vi "Read Config File.vi"(7 "LabVIEW Dir Override":path, 8 "error in (no error)":errorcluster, 10 "Config File In":string, 11 "Project Source Root":path) -> (0 "error out":errorcluster, 3 "Configuration out":T1)   [LabVIEW 2011, in "LVH-Build-Tools.lvlib"]
uses:
  LVH-Build-Tools.lvlib
  Type Defs/Configuration.ctl
  Type Defs/Install Configuration.ctl
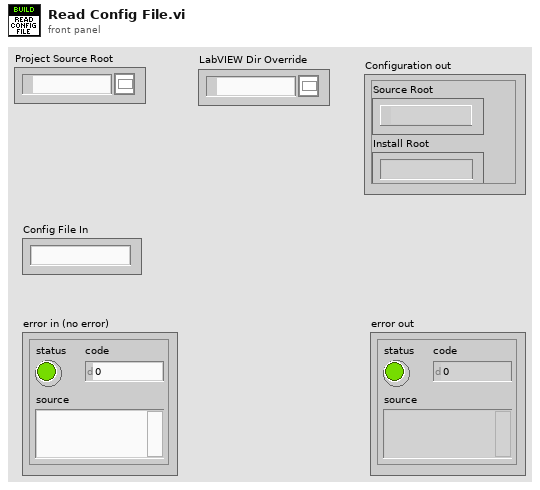
[diagram p1: front panel]
types:
  T1 = typedef "LVH-Build-Tools.lvlib/Configuration.ctl" = cluster{"Source Root":path, "Install Root":string, "Components":string[], "Ignore":string[], "Config Files":path[], "LV Directories":path[], "Install Paths":T2}
  T2 = typedef "LVH-Build-Tools.lvlib/Install Configuration.ctl" = cluster{"LabVIEW Directory":path, "Project Source Config":path}
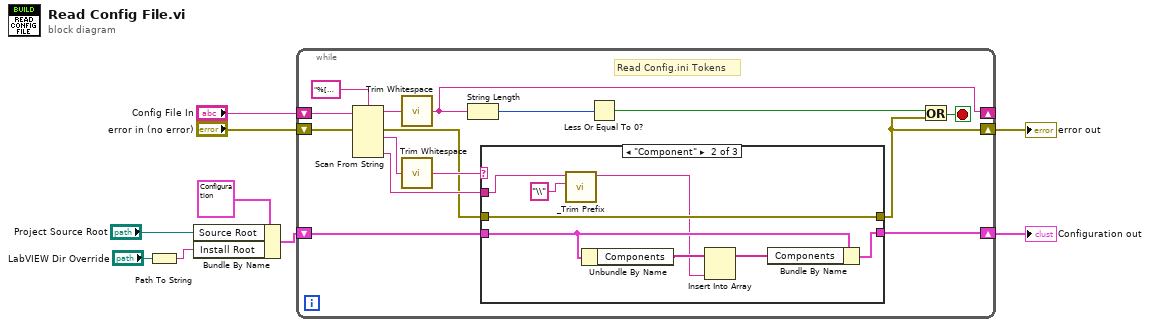
[diagram p0: block diagram]
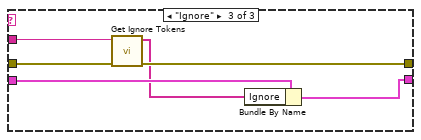
[diagram p3: hidden frame]
diagram:
  n1 = Path To String(path="LabVIEW Dir Override") -> (string=w1:string)
  n2 = Bundle By Name(cluster=T1 {"Source Root"=path "", "Install Root"="", "Components"=[], "Ignore"=[], "Config Files"=[], "LV Directories"=[], "Install Paths"={"LabVIEW Directory"=path "", "Project Source Config"=path ""}} ("Configuration in"), "Source Root"="Project Source Root", "Install Root"=w1) -> (w4:T1)
  n3 = while {
    shift-right: [w14] -> _
    shift-left: "Config File In" -> [w23]
    shift-right: [w12] -> w8
    shift-left: "error in (no error)" -> [w22]
    shift-right: [w10] -> w9
    shift-left: w4 -> [w11]
    stop <- w18 stop-if-true
    # "Read Config.ini Tokens"
    n4 = Scan From String(format string="%[^=] %[=] %[^\n]", input string=w23, error in=w22) -> (remaining string=w15:string, error out=w13:errorcluster, output 1=w17:string, output 3=w20:string)  [unwired: 5 in, 1 out]
    n5 = call <vilib>:"Trim Whitespace.vi"("string"=w15) -> ("trimmed string"=w14:string)  [unwired: 1 in]
    n6 = call <vilib>:"Trim Whitespace.vi"("string"=w17) -> ("trimmed string"=w16:string)  [unwired: 1 in]
    n7 = String Length(string=w14) -> (length=w21:i32)
    n8 = case shown="\"Component\"" w16 {
      tunnel: w20 -> [_ w29 w40]
      tunnel: w13 -> [w26 w34 w39]
      tunnel: [w26 w34 w38] -> w12
      tunnel: [w25 w30 w36] -> w10
      tunnel: w11 -> [w25 w33 w37]
      frame Default {
      }
      frame "Component" {
        n9 = call "_Trim Prefix.vi"("Prefix"="\\", "String"=w29) -> ("String"=w27:string)  [unwired: 9 in]
        n10 = Unbundle By Name(w33) -> ("Components"=w32:string[])
        n11 = Insert Into Array(array=w32, new element=w27) -> (w31:string[])  [unwired: 1 in]
        n12 = Bundle By Name(cluster=w33, "Components"=w31) -> (w30:T1)
      }
      frame "Ignore" {
        n13 = call "Get Ignore Tokens.vi"("Error In"=w39, "Ignore String"=w40) -> ("ErrorOut"=w38:errorcluster, "Ignore Tokens"=w35:string[])  [unwired: 8 in]
        n14 = Bundle By Name(cluster=w37, "Ignore"=w35) -> (w36:T1)
      }
    }
    n15 = Less Or Equal To 0?(x=w21) -> (x <= 0?=w19:bool)
    n16 = Or(x=w19, y=w12) -> (x .or. y?=w18:bool)
  }
  "Configuration out" <- w9
  "error out" <- w8
